vi "Kei237_Set_Voltage_488-2.vi"(0 "Voltage":dbl format="%.3p", 1 "GPIB Address":i8=16) -> ()   [LabVIEW 2009]
panel:
  # "Keithley 237 Set Voltage"
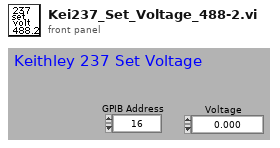
[diagram p1: front panel]
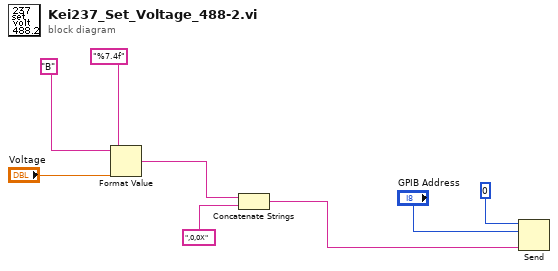
[diagram p0: block diagram]
diagram:
  n1 = Format Value(string ("")="B", format string="%7.4f", value (0)="Voltage") -> (output string=w2:string)
  n2 = Concatenate Strings(w2, ",0,0X") -> (w1:string)
  n3 = Send(0:0, 2:"GPIB Address", 5:w1) -> ()  [unwired: 2 in, 3 out]
